vi "OAT Even Time or Speed Segment (Even Angle, 1 Channel).vi"(0 "even-angle signal":cluster{"r0":dbl, "dr":dbl, "Y":dbl[]}={"r0"=0.0, "dr"=1.0, "Y"=[]} {"r0" format="%.2p"; "dr" format="%.2p"; "Y" format="%.2f"}, 1 "segment unit":u16(ring) items=["Time (s)", "Speed (RPM)"], 2 "reset? (F)":bool, 5 "even-angle channel info":T2={"channel name"="", "description"="", " channel info"={"sensor sensitivity"=1000.0, "engineering units"=1, "dB reference"=1.0, "custom label"="EU", "weighting filter"=0, "pregain"=0.0}} {"channel info"."pregain" format="%.2f"; "channel info"."weighting filter" items=["Linear", "A-weighting", "B-weighting", "C-weighting", "ITU-R 468-4", "Dolby", "CCITT", "C-message", "Wb", "Wc", "Wd", "We", "Wf", "Wh", "Wj", "Wk", "Wm", "AES17 20 kHz lowpass", "AES17 40 kHz lowpass", "AES17 20 kHz highpass", "AES17 40 kHz highpass"]; "channel info"."dB reference" format="%^.1e"; "channel info"."engineering units" items=["custom..."=0, "V"=1, "A"=21, "C"=30, "pC"=31, "s"=32, "-"=29, "Pa"=2, "N"=20, "g"=3, "m/s^2"=4, "m/s"=5, "m"=6, "mm/s"=12, "mm"=13, "micron/s"=14, "micron"=15, "in/s^2"=7, "in/s"=8, "in"=9, "mil/s"=10, "mil"=11, "rad/s^2"=16, "rad/s"=17, "rad"=18, "deg/s^2"=26, "deg/s"=27, "deg"=28, "RPM"=22, "cycle/s^2"=23, "Hz"=24, "cycle"=25, "strain"=19]; "channel info"."sensor sensitivity" format="%#_5f"}, 7 "speed profile":T7 {"speed [RPM]" format="%.2f"; "time [s]" format="%.2f"}, 9 "pulse/revolution (1)":i32=1, 11 "error in (no error)":errorcluster, 12 "segment settings":cluster{"start":dbl, "end":dbl, "step size":dbl} {"step size" format="%.2f"; "end" min=0.0 format="%.2f"; "start" min=0.0 format="%.2f"}, 13 "segment block size":i32=128 min=2) -> (4 "even-angle signal out":cluster{"r0":dbl, "dr":dbl, "Y":dbl[]}={"r0"=0.0, "dr"=1.0, "Y"=[]} {"r0" format="%.2p"; "dr" format="%.2p"; "Y" format="%.2f"}, 6 "dup even-angle channel info":T2={"channel name"="", "description"="", " channel info"={"sensor sensitivity"=1000.0, "engineering units"=1, "dB reference"=1.0, "custom label"="EU", "weighting filter"=0, "pregain"=0.0}} {"channel info"."pregain" format="%.2f"; "channel info"."weighting filter" items=["Linear", "A-weighting", "B-weighting", "C-weighting", "ITU-R 468-4", "Dolby", "CCITT", "C-message", "Wb", "Wc", "Wd", "We", "Wf", "Wh", "Wj", "Wk", "Wm", "AES17 20 kHz lowpass", "AES17 40 kHz lowpass", "AES17 20 kHz highpass", "AES17 40 kHz highpass"]; "channel info"."dB reference" format="%^.1e"; "channel info"."engineering units" items=["custom..."=0, "V"=1, "A"=21, "C"=30, "pC"=31, "s"=32, "-"=29, "Pa"=2, "N"=20, "g"=3, "m/s^2"=4, "m/s"=5, "m"=6, "mm/s"=12, "mm"=13, "micron/s"=14, "micron"=15, "in/s^2"=7, "in/s"=8, "in"=9, "mil/s"=10, "mil"=11, "rad/s^2"=16, "rad/s"=17, "rad"=18, "deg/s^2"=26, "deg/s"=27, "deg"=28, "RPM"=22, "cycle/s^2"=23, "Hz"=24, "cycle"=25, "strain"=19]; "channel info"."sensor sensitivity" format="%#_5f"}, 8 "new signal available?":bool, 10 "current segment status":T6, 14 "actual segment settings":T1 {"actual step size" format="%.2f"; "actual end" min=0.0 format="%.2f"; "actual start" min=0.0 format="%.2f"}, 15 "error out":errorcluster)   [LabVIEW 2017, in "SoundVib_OAUtility.lvlib"]
doc: "Divides an input signal into even-time segments or even-speed intervals. The input signal of this VI can be an even-angle signal or an XY signal. When you use this VI to divide an XY signal, the XY signal can be only the output of the OAT Order Magnitude and Phase VI or OAT Overall Level Plot VI. Wire data to the <B>even-angle signal</B> input to determine the polymorphic instance to use or manually select the instance."
uses:
  <vilib>/addons/Sound and Vibration/Order Analysis/Utility/SoundVib_OAUtility.lvlib
  <vilib>/addons/_NISVFA/_Shared subVIs/Controls/svc_Resampled Channel Info.ctl
  <vilib>/addons/_NISVFA/_Shared subVIs/Controls/svc_Channel Info.ctl
  <vilib>/addons/_NISVFA/_Shared subVIs/Controls/svc_Engineering Units Text Ring.ctl
  <vilib>/addons/_NISVFA/_Shared subVIs/Controls/svc_Weighting Filter Text Ring.ctl
  <vilib>/addons/Sound and Vibration/Order Analysis/Tach Process/SubVIs/speed profile.ctl
  <vilib>/addons/Sound and Vibration/Order Analysis/Tach Process/SoundVib_TachProcess.lvlib
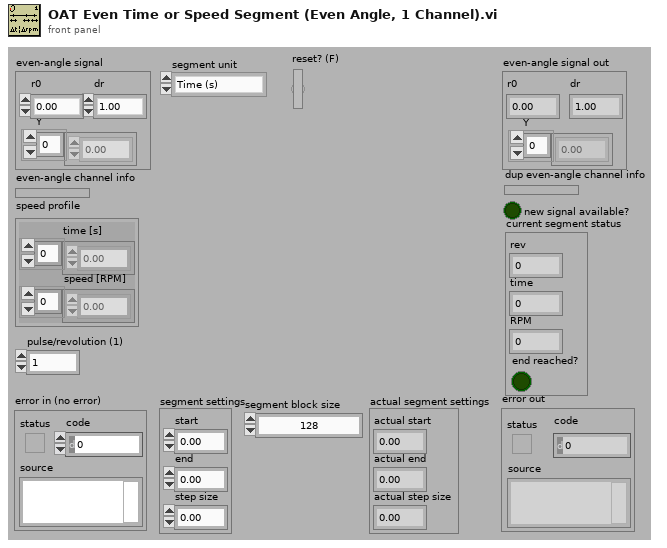
[diagram p1: front panel]
types:
  T1 = cluster{"actual start":dbl, "actual end":dbl, "actual step size":dbl}
  T2 = typedef "svc_Resampled Channel Info.ctl" = cluster{"channel name":string, "description":string, " channel info":T3}
  T3 = typedef "svc_Channel Info.ctl" = cluster{"sensor sensitivity":dbl, "engineering units":T4, "dB reference":dbl, "custom label":string, "weighting filter":T5, "pregain":dbl}
  T4 = typedef "svc_Engineering Units Text Ring.ctl" = u16
  T5 = typedef "svc_Weighting Filter Text Ring.ctl" = u16
  T6 = cluster{"rev":dbl, "time":dbl, "RPM":dbl, "end reached?":bool}
  T7 = typedef "SoundVib_TachProcess.lvlib/speed profile.ctl" = cluster{"time [s]":dbl[], "speed [RPM]":dbl[]}
  T8 = cluster{"rev":dbl, "time":dbl, "RPM":dbl, "finish?":bool}
  T9 = cluster{"last rev":dbl, "rev indice":dbl[], "time indice":dbl[], "RPM indice":dbl[]}
  T10 = cluster{"rev":dbl, "time":dbl, "RPM":dbl, "reached end?":bool}
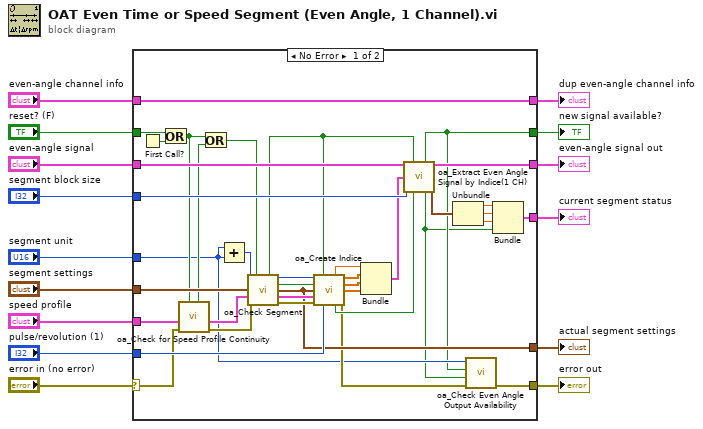
[diagram p0: block diagram]
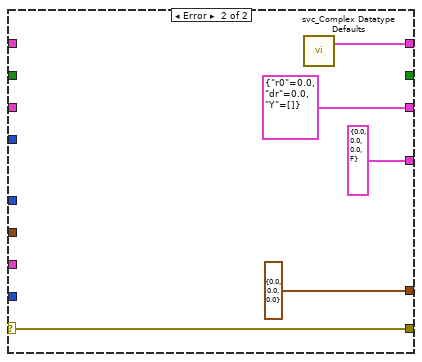
[diagram p2: hidden frame]
diagram:
  n1 = case shown="No Error" "error in (no error)" {
    selector: "error in (no error)" -> [w22 w58]
    tunnel: [w19 w58] -> w2
    tunnel: "reset? (F)" -> [w29 _]
    tunnel: "segment unit" -> [w18 _]
    tunnel: "segment settings" -> [w35 _]
    tunnel: "speed profile" -> [w34 _]
    tunnel: "even-angle channel info" -> [w53 _]
    tunnel: [w53 w55] -> w6
    tunnel: [w33 cluster{"start":dbl, "end":dbl, "step":dbl} {"start"=0.0, "end"=0.0, "step"=0.0} ("steps output")] -> w3
    tunnel: "pulse/revolution (1)" -> [w52 _]
    tunnel: "segment block size" -> [w51 _]
    tunnel: "even-angle signal" -> [w50 _]
    tunnel: [w44 cluster{"r0":dbl, "dr":dbl, "Y":dbl[]} {"r0"=0.0, "dr"=0.0, "Y"=[]} ("even angle signal output")] -> w5
    tunnel: [w39 T8 {"rev"=0.0, "time"=0.0, "RPM"=0.0, "finish?"=FALSE} ("current segment position")] -> w4
    tunnel: [w17 _] -> w1
    frame No Error {
      n2 = First Call?() -> (First Call?: T/F=w30:bool)
      n3 = Or(x=w29, y=w30) -> (x .or. y?=w25:bool)
      n4 = call <vilib>:"oa_Check for Speed Profile Continuity.vi"("reset in"=w25, "error in (no error)"=w22, "speed profile"=w34) -> ("error out"=w21:errorcluster, "speed profile dup"=w26:T7, "position not continuous"=w23:bool)  [unwired: 6 in]
      n5 = Or(x=w25, y=w23) -> (x .or. y?=w24:bool)
      n6 = Add(x=w18, y=w18) -> (x+y=w31:u16)
      n7 = call <vilib>:"oa_Check Segment.vi"("X axis selection"=w31, "reset?(F)"=w24, "segment position"=w35, "speed profile"=w26, "error in (no error)"=w21) -> ("reset out"=w27:bool, "X axis selection"=w32:u16, "step found?"=w38:bool, "segment position out"=w33:cluster{"start":dbl, "end":dbl, "step size":dbl}, "dul speed profile"=w37:T7, "error out"=w36:errorcluster)  [unwired: 5 in]
      n8 = call <vilib>:"oa_Create Indice.vi"("X axis selection"=w32, "reset?(F)"=w27, "step found?(F)"=w38, "steps input"=w33, "speed profile"=w37, "error in (no error)"=w36, "pulse/revolution (1)"=w52) -> ("last rev"=w49:dbl, "rev indice"=w48:dbl[], "time indice"=w47:dbl[], "RPM indice"=w46:dbl[], "reach end?"=w28:bool, "error out"=w20:errorcluster)  [unwired: 2 in, 1 out]
      n9 = Bundle("last rev"=w49, "rev indice"=w48, "time indice"=w47, "RPM indice"=w46) -> (w45:T9)  [unwired: 1 in]
      n10 = call <vilib>:"oa_Extract Even Angle Signal by Indice(1 CH).vi"("even angle signal"=w50, "reset?"=w27, "trigger indices"=w45, "block size"=w51, "indices end?"=w28) -> ("new signal available?"=w17:bool, "even angle signal output"=w44:cluster{"r0":dbl, "dr":dbl, "Y":dbl[]}, "reached end?"=w16:bool, "current positon"=w43:cluster{"rev":dbl, "time":dbl, "RPM":dbl})  [unwired: 7 in]
      n11 = Unbundle(w43) -> ("rev"=w42:dbl, "time"=w41:dbl, "RPM"=w40:dbl)
      n12 = call <vilib>:"oa_Check Even Angle Output Availability.vi"("error in (no error)"=w20, "reached end?"=w16, "new signal available?"=w17, "segment unit"=w18) -> ("error out"=w19:errorcluster)  [unwired: 7 in]
      n13 = Bundle("rev"=w42, "time"=w41, "RPM"=w40, "reached end?"=w16) -> (w39:T10)  [unwired: 1 in]
    }
    frame Error {
      n14 = call <vilib>:"svc_Complex Datatype Defaults.vi"() -> ("resampled channel info"=w55:T2)  [unwired: 11 in, 8 out]
    }
  }
  "error out" <- w2
  "even-angle signal out" <- w5
  "current segment status" <- w4
  "dup even-angle channel info" <- w6
  "actual segment settings" <- w3
  "new signal available?" <- w1
